vi "Gyro PID Fwd Color Assisted.vi"(6 "Target angle":sgl, 7 "Threshold to Color":i32=1200, 8 "Threshold to slow":i32=1000, 9 "Min. speed":i32=40, 10 "Max. speed":i32=80, 11 "EV3 in":T1) -> (3 "EV3 out":T1)   [LabVIEW 2015]
uses:
  <vilib>/NXT/Block Support/NXT_OutputPort.ctl
  <vilib>/NXT/LegoClasses/BrickReference/BrickReference.lvclass
  <vilib>/NXT/Subs/LVHSConnector.ctl
  <vilib>/NXT/NXTIO Xnodes/NXTIONodeSubVIs/NXTMotorSteeringOn.vi
  <vilib>/NXT/NXTIO Xnodes/NXTIOXNode/NXTIO.xnode
  <vilib>/NXT/NXTIO Xnodes/NXTIONodeSubVIs/LEGOResetMotors.vi
  <vilib>/NXT/NXTIO Xnodes/NXTIONodeSubVIs/NXTStopMotors.vi
  <vilib>/NXT/Dual Mode Library/Motors/Rotation.vi
  <vilib>/NXT/Block Support/NXT_InputPort.ctl
  <vilib>/NXT/Dual Mode Library/Sensors/EV3_Color_Reflect.vi
  <vilib>/NXT/Dual Mode Library/Waits/Wait_Num.vi
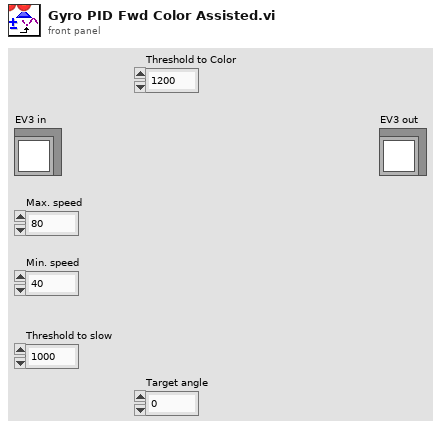
[diagram p1: front panel]
types:
  T1 = typedef "LVHSConnector.ctl" = refnum<class "BrickReference.lvclass">
  T2 = typedef "NXT_OutputPort.ctl" = u8
  T3 = typedef "NXT_InputPort.ctl" = u32
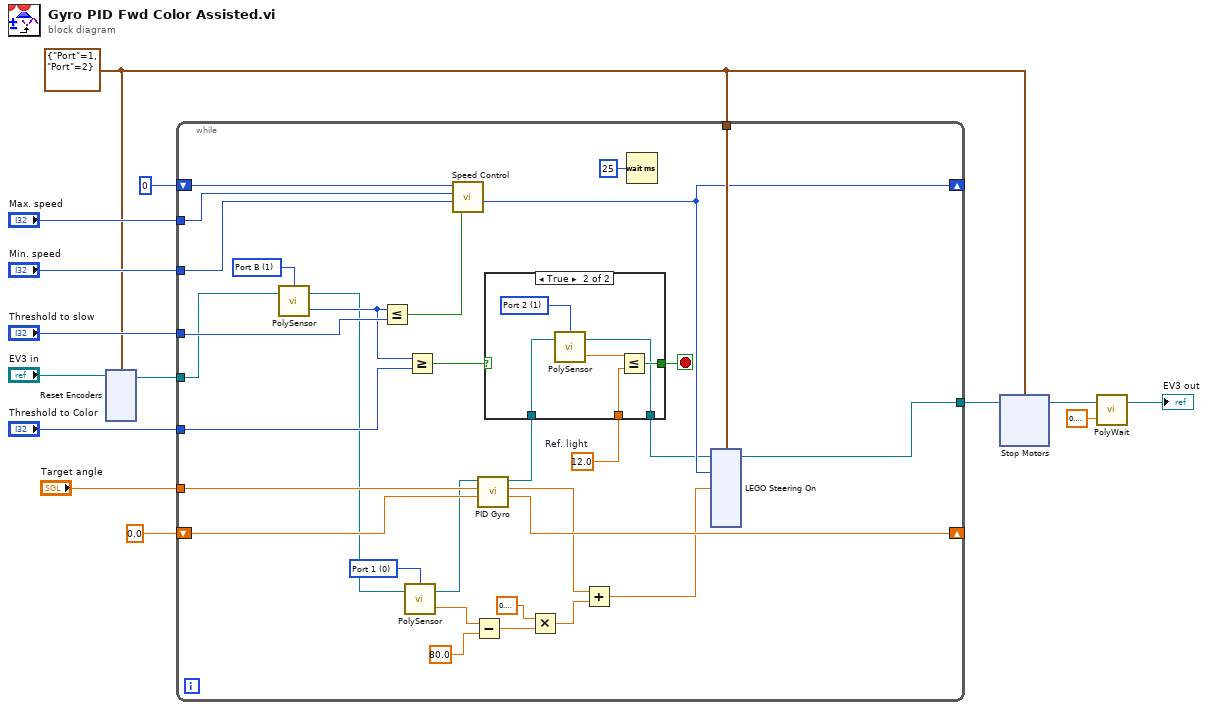
[diagram p0: block diagram]
diagram:
  w4 = cluster{"Port":T2, "Port":T2} {"Port"=1, "Port"=2} ("Motor")
  n1 = xnode "Reset Encoders"("Motors"=w4, "NXT/EV3"="EV3 in") -> ("NXT/EV3"=w10:T1)
  n2 = while {
    tunnel: w10 -> [w35]
    shift-right: [w45] -> _
    shift-left: sgl 0.0 -> [w32]
    tunnel: "Target angle" -> [w44]
    tunnel: [w41] -> w6
    tunnel: w4 -> [w43]
    shift-right: [w31] -> _
    shift-left: 0 -> [w39]
    tunnel: "Min. speed" -> [w36]
    tunnel: "Max. speed" -> [w38]
    tunnel: "Threshold to slow" -> [w37]
    tunnel: "Threshold to Color" -> [w30]
    stop <- w29 stop-if-true
    w24 = T3 0 items=["Port 1", "Port 2", "Port 3", "Port 4"] ("Port (Port 1)")
    w25 = sgl 12.0  # Ref. light
    w42 = T2 1 items=["Port A", "Port B", "Port C", "Port D"] ("Port (Port A)")
    n3 = call-poly <vilib>:"PolySensor.vi"("NXT/EV3"=w35, "Port (Port A)"=w42) -> ("Angle of Rotation"=w33:i32, "NXT/EV3"=w22:T1)  [unwired: 1 in]
    n4 = Less Or Equal?(x=w33, y=w37) -> (x <= y?=w34:bool)
    n5 = call-poly <vilib>:"PolySensor.vi"("NXT/EV3"=w22, "Port (Port 1)"=w24) -> ("Scaled Value"=w23:sgl, "NXT/EV3"=w21:T1)  [unwired: 1 in]
    n6 = Greater Or Equal?(x=w33, y=w30) -> (x >= y?=w28:bool)
    n7 = call "Speed Control.vi"("Speed Up or Down?"=w34, "Min. speed"=w36, "Max. speed"=w38, "Ini. speed"=w39) -> ("Speed out"=w31:i32)  [unwired: 7 in]
    n8 = Subtract(x=w23, y=sgl 80.0) -> (x-y=w19:sgl)
    n9 = call "PID Gyro.vi"("Previous integral"=w32, "Target angle"=w44, "EV3 in"=w21) -> ("New integral"=w45:sgl, "Total error"=w16:sgl, "EV3 out"=w27:T1)  [unwired: 6 in]
    n10 = case shown="True" w28 {
      tunnel: [_ w50] -> w29
      tunnel: w27 -> [w46 w49]
      tunnel: [w46 w48] -> w26
      tunnel: w25 -> [_ w47]
      frame False {
      }
      frame True {
        w52 = T3 1 items=["Port 1", "Port 2", "Port 3", "Port 4"] ("Port (Port 1)")
        n11 = call-poly <vilib>:"PolySensor.vi"("NXT/EV3"=w49, "Port (Port 1)"=w52) -> ("Scaled Value"=w51:sgl, "NXT/EV3"=w48:T1)  [unwired: 1 in]
        n12 = Less Or Equal?(x=w51, y=w47) -> (x <= y?=w50:bool)
      }
    }
    n13 = Multiply(x=sgl 0.1, y=w19) -> (x*y=w17:sgl)
    n14 = Add(x=w16, y=w17) -> (x+y=w15:sgl)
    n15 = Wait (ms)(milliseconds to wait=u32 25) -> ()  [unwired: 1 out]
    n16 = xnode "LEGO Steering On"("Steering 1"=w15, "Power 1"=w31, "Motors"=w43, "NXT/EV3"=w26) -> ("NXT/EV3"=w41:T1)
  }
  n17 = xnode "Stop Motors"("Motors"=w4, "NXT/EV3"=w6) -> ("NXT/EV3"=w5:T1)
  n18 = call-poly <vilib>:"PolyWait.vi"("Time (1 sec)"=sgl 0.2, "NXT/EV3"=w5) -> ("NXT/EV3"=→"EV3 out":T1)  [unwired: 2 in]
